vi "SendIntTime.vi"(3 "error in (no error)":errorcluster, 5 "Instruments in":refnum<class "Instruments.lvclass">) -> (0 "error out":errorcluster, 1 "IntTime":i32, 2 "Instruments out":refnum<class "Instruments.lvclass">)   [LabVIEW 2012, in "Instruments.lvclass"]
uses:
  Instruments.lvclass
  Instruments.lvclass/Instruments.ctl
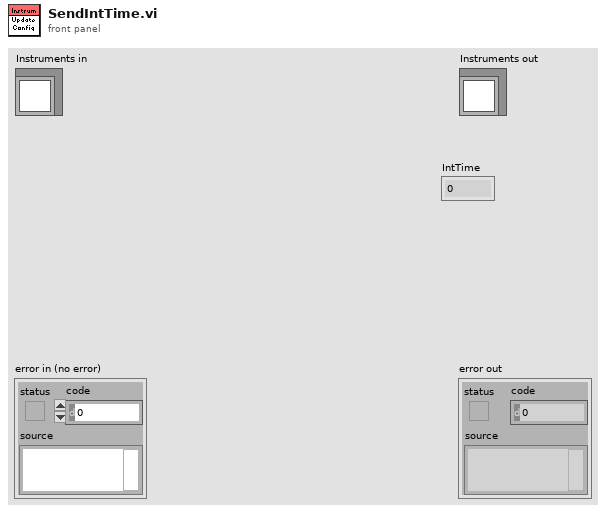
[diagram p1: front panel]
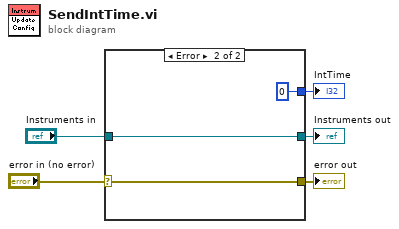
[diagram p0: block diagram]
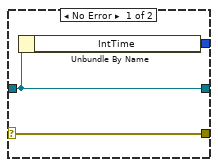
[diagram p2: hidden frame]
diagram:
  n1 = case shown="Error" "error in (no error)" {
    selector: "error in (no error)" -> [w8 w9]
    tunnel: [w8 w9] -> w4
    tunnel: [w6 w11] -> w2
    tunnel: "Instruments in" -> [w6 w11]
    tunnel: [w7 0 ("IntTime")] -> w1
    frame No Error {
      n2 = Unbundle By Name(w6) -> ("IntTime"=w7:i32)
    }
    frame Error {
    }
  }
  "error out" <- w4
  "Instruments out" <- w2
  "IntTime" <- w1
